vi "Test Latch until released.vi"(11 "Error in":errorcluster) -> (15 "Error out":errorcluster)   [LabVIEW 2020, in "Mechanical Actions Tests.lvlib"]
doc: "This VI is used to test latch untill release function"
uses:
  Mechanical Actions Tests.lvlib
  <vilib>/addons/_JKI Toolkits/Caraya/classes/Test Suite/Define Test Suite (JUnit Report).vi
  <vilib>/SLL Drona/APIs/Stimulus/ControlValue/SetValueAuto.vi
  <vilib>/SLL Drona/APIs/Assert/AssertControlValue/Less.vi
  <vilib>/SLL Drona/APIs/Assert/AssertControlValue/Equal.vi
  <vilib>/SLL Drona/APIs/Stimulus/VI/CloseVI.vi
  <vilib>/Utility/error.llb/Error Cluster From Error Code.vi
  <vilib>/ErrorRing/Error Ring.xnode
  <vilib>/addons/_JKI Toolkits/Caraya/classes/Test Suite/Test Suite.lvclass
  <vilib>/SLL Drona/Drona.lvlib
  <vilib>/SLL Drona/APIs/Stimulus/ControlValue/ControlValue.lvlib
  <vilib>/SLL Drona/APIs/Assert/AssertControlValue/AssertControlValue.lvlib
  <vilib>/addons/_JKI Toolkits/Caraya/classes/Test/Test.lvclass
  <vilib>/Wiresmith Technology/G CLI/CLI Class/CLI.lvclass
  <vilib>/SLL Drona/APIs/Stimulus/VI/VI.lvlib
panel:
  # "LATCH UNTILL RELEASE TEST"
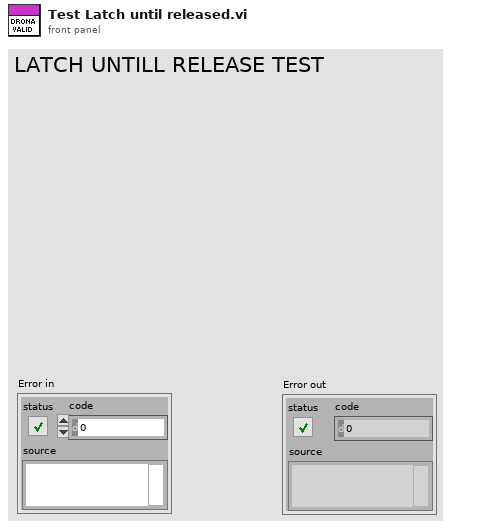
[diagram p1: front panel]
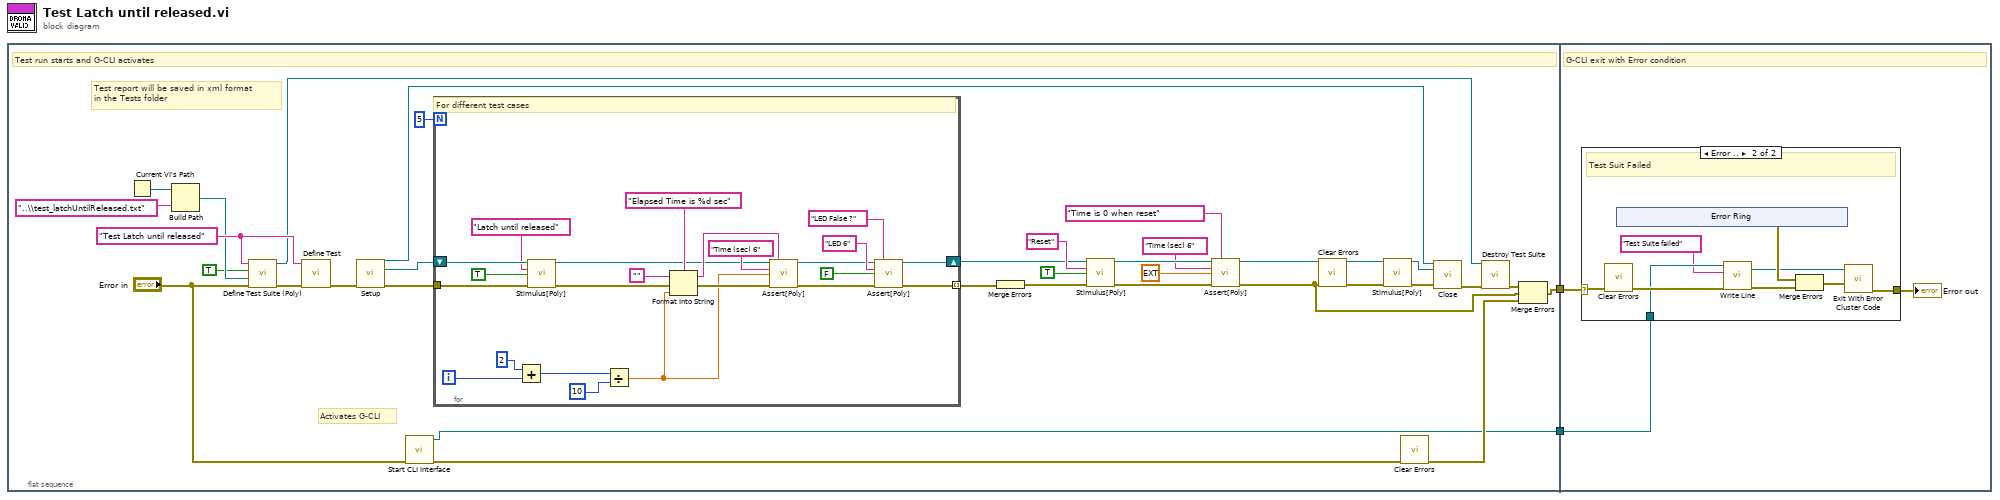
[diagram p0: block diagram]
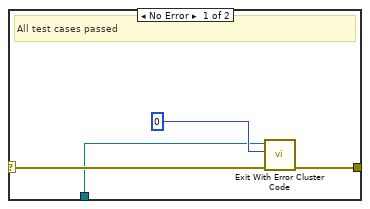
[diagram p2: hidden frame]
diagram:
  n1 = flat-sequence {
    tunnel: [w18] -> w2
    tunnel: [w5] -> w1
    tunnel: w2 -> [w62]
    tunnel: w1 -> [w60]
    frame #0 {
      w14 = "Test Latch until released" ("Label (VI Title)")
      # "Test report will be saved in xml format\nin the Tests folder"
      # "Activates G-CLI"
      # "Test run starts and G-CLI activates"
      n2 = Current VI's Path() -> (path=w13:path)
      n3 = Build Path(base path=w13, name or relative path="..\\test_latchUntilReleased.txt") -> (appended path=w11:path)
      n4 = call-poly <vilib>:"Define Test Suite (Poly).vi"("error in (no error)"="Error in", "Report Path"=w11, "Interactive"=TRUE, "Label (VI Title)"=w14) -> ("error out"=w16:errorcluster, "Test Suite"=w7:refnum<class "Test Suite.lvclass">)  [unwired: 5 in, 1 out]
      n5 = call <vilib>:"Define Test.vi"("error in (no error)"=w16, "Label (VI Title)"=w14) -> ("error out"=w36:errorcluster)  [unwired: 8 in, 1 out]
      n6 = call <vilib>:"Setup.vi"("error in"=w36) -> ("Application Ref"=w25:refnum<vi>, "VI Reference Out"=w35:refnum<vi>, "error out"=w23:errorcluster)  [unwired: 12 in]
      n7 = call <vilib>:"Start CLI Interface.vi"("error in (no error)"="Error in") -> ("error out"=w6:errorcluster, "CLI out"=w5:refnum<class "CLI.lvclass">)  [unwired: 7 in, 2 out]
      n8 = for {
        N: 5 -> [_]
        shift-right: [w41] -> w27
        shift-left: w35 -> [w58]
        tunnel: w23 -> [w59]
        tunnel: [w42] -> w26 mode=indexing
        i -> [w51]
        # "For different test cases"
        n9 = Add(x=2, y=w51) -> (x+y=w38:i32)
        n10 = call-poly <vilib>:"Stimulus[Poly].vi"("VI Reference In"=w58, "Control Path"="Latch until released", "Value (Signaling)"=TRUE, "error in"=w59) -> ("VI Reference Out"=w45:refnum<vi>, "error out"=w46:errorcluster)  [unwired: 10 in]
        n11 = Divide(x=w38, y=10) -> (x/y=w39:dbl)
        n12 = Format Into String(format string="Elapsed Time is %d sec", initial string="", error in=w46, w39) -> (resulting string=w47:string, error out=w50:errorcluster)
        n13 = call-poly <vilib>:"Assert[Poly].vi"("VI Reference In"=w45, "Test Label"=w47, "Control Path"="Time (sec) 6", "Control Value"=w39, "Error In"=w50) -> ("VI Reference Out"=w44:refnum<vi>, "Error Out"=w43:errorcluster)  [unwired: 9 in]
        n14 = call-poly <vilib>:"Assert[Poly].vi"("VI Reference In"=w44, "Test Label"="LED False ?" ("Label"), "Control Path"="LED 6", "Control Value"=FALSE, "Error In"=w43) -> ("VI Reference Out"=w41:refnum<vi>, "Error Out"=w42:errorcluster)  [unwired: 9 in]
      }
      n15 = Merge Errors(w26) -> (w24:errorcluster)
      n16 = call-poly <vilib>:"Stimulus[Poly].vi"("VI Reference In"=w27, "Control Path"="Reset", "Value (Signaling)"=TRUE, "error in"=w24) -> ("VI Reference Out"=w34:refnum<vi>, "error out"=w33:errorcluster)  [unwired: 10 in]
      n17 = call-poly <vilib>:"Assert[Poly].vi"("VI Reference In"=w34, "Test Label"="Time is 0 when reset" ("Label"), "Control Path"="Time (sec) 6", "Control Value"=ext 0.0, "Error In"=w33) -> ("VI Reference Out"=w21:refnum<vi>, "Error Out"=w3:errorcluster)  [unwired: 9 in]
      n18 = call <vilib>:"Clear Errors.vi"("error in (no error)"=w3) -> ("error out"=w4:errorcluster)  [unwired: 5 in, 1 out]
      n19 = call-poly <vilib>:"Stimulus[Poly].vi"("VI Reference In"=w21, "error in"=w4) -> ("VI Reference Out"=w20:refnum<vi>, "error out"=w19:errorcluster)  [unwired: 12 in]
      n20 = call <vilib>:"Clear Errors.vi"("error in (no error)"=w6) -> ("error out"=w17:errorcluster)  [unwired: 5 in, 1 out]
      n21 = call <vilib>:"Close.vi"("Application Ref"=w25, "VI Reference"=w20, "error in"=w19) -> ("error out"=w9:errorcluster)  [unwired: 12 in]
      n22 = call-dynamic "Destroy Test Suite.vi"("error in (no error)"=w9, "Test Suite in"=w7) -> ("error out"=w8:errorcluster)  [unwired: 8 in, 1 out]
      n23 = Merge Errors(w8, w3, w17) -> (w18:errorcluster)
    }
    frame #1 {
      # "G-CLI exit with Error condition"
      n24 = case shown="Error .." w62 {
        selector: w62 -> [w66 w74]
        tunnel: [w65 w75] -> w61
        tunnel: w60 -> [w63 w72]
        frame No Error {
          # "All test cases passed"
          n25 = call <vilib>:"Exit With Error Cluster Code.vi"("error in (no error)"=w66, "No Error Code (0)"=0, "CLI in"=w63) -> ("error out"=w65:errorcluster)  [unwired: 8 in]
        }
        frame Error {
          # "Test Suit Failed"
          n26 = call <vilib>:"Clear Errors.vi"("error in (no error)"=w74) -> ("error out"=w73:errorcluster)  [unwired: 5 in, 1 out]
          n27 = xnode "Error Ring"() -> ("error out"=w69:errorcluster)
          n28 = call <vilib>:"Write Line.vi"("error in (no error)"=w73, "Text to Write"="Test Suite failed", "CLI in"=w72) -> ("error out"=w68:errorcluster, "CLI out"=w67:refnum<class "CLI.lvclass">)  [unwired: 7 in]
          n29 = Merge Errors(w69, w68) -> (w70:errorcluster)
          n30 = call <vilib>:"Exit With Error Cluster Code.vi"("error in (no error)"=w70, "CLI in"=w67) -> ("error out"=w75:errorcluster)  [unwired: 9 in]
        }
      }
      "Error out" <- w61
    }
  }
